vi "Single Slow IV v1.8.vi"() -> ()   [LabVIEW 2023]
uses:
  <vilib>/Utility/file.llb/Write Delimited Spreadsheet (DBL).vi
panel:
  out "Current variable":dbl=-0.010000000000000009
  in  "stop":bool
  in  "Tab Control 2":T1(tab)
  out "cRIO data plot":cluster{"Y":dbl[], "Y":dbl[]}[](graph)
  out "cRIO Plot 0":string="DC Voltage V"
  out "cRIO Plot 1":string="DC current uA"
  out "cRIO Plot 2":string="dV V"
  out "cRIO Plot 3":string="dI uA"
  out "Lockin X":cluster{"Y":dbl[], "Y":dbl[]}[](graph)
  out "Lockin Y":cluster{"Y":dbl[], "Y":dbl[]}[](graph)
  in  "Tab Control":T2(tab)
  out "Unit":string="uA"
  in  "Tab for variable":enum32{"Current", "Magnetic field"}(tab)
  in  "Delay Time s":dbl=0.1 caption="Delay Time (s)"
  in  "AO Channel":string(combo)="AO0"
  in  "current output Scale factor":dbl=1.0
  in  "Fixed current uA":dbl=2.1
  in  "Scale factor":dbl=1.0
  in  "Field Rate mT per sec":dbl=0.1 format="%#_13g"
  in  "Magnet Device Select":string(combo)="NI DAQ Controlled V to I source"
  in  "Start":dbl
  in  "Range":dbl=1.0
  in  "Step":dbl=0.01
  in  "Ramp type":string(combo)="Around origin"
  in  "Ramp up first T":bool=TRUE
  in  "cRIO Chan 0":bool=TRUE
  in  "cRIO IP":string="//172.22.11.2"
  in  "Reading Average times":i32=100
  in  "read cRIO":bool=TRUE
  in  "Scale factor3":dbl=1.0
  in  "Channel name 3":string(combo)="dI uA"
  in  "cRIO Chan 3":bool
  in  "Scale factor2":dbl=1.0
  in  "Channel name 2":string(combo)="dV V"
  in  "cRIO Chan 2":bool
  in  "Scale factor1":dbl=1.0
  in  "Channel name 1":string(combo)="DC current uA"
  in  "cRIO Chan 1":bool=TRUE
  in  "Scale factor0":dbl=0.0001
  in  "Channel name 0":string(combo)="DC Voltage V"
  in  "Lockin address 4":string
  in  "Lockin address 3":string
  in  "Lockin address 2":string="GPIB0::9::INSTR"
  in  "Lockin address 1":string="GPIB0::8::INSTR"
  in  "Lockin 4":bool
  in  "Lockin 3":bool
  in  "Lockin 2":bool
  in  "Lockin 1":bool
  in  "Use Lockin":bool
  in  "Lockin Chan name 4":string(combo)="None"
  in  "Lockin Chan name 3":string(combo)="None"
  in  "Lockin Chan name 2":string(combo)="Current mV"
  in  "Lockin Chan name 1":string(combo)="Voltage mV"
  out "DAQ_CMD_Writer endpoint":refnum<k21>="DAQ_CMD_Writer"
  out "DAQ_AI_Reader endpoint":refnum<k21>="DAQ_AI_Reader"
  in  "Lockin and field and temperature status":string="Data File time stamp 20230818-143806\nTemperature Chan1 1.218210, Chan2 0.069148\nmagnetic field InfmT\nLockin status\n"
  in  "Temp Device":string(combo)="Elsa"
  in  "Temp Chan1":string="T5"
  in  "Temp Chan2":string="T8"
  in  "Magnetic field read device":string(combo)="None"
  in  "Record Field":bool
  out "error out":errorcluster
  in  "Contour plot folder":path=path "C:/Users/gyue/Desktop/20230814 Soorya devices"
  # "NOTE:  Tab pressed below change output signal"
  # "Voltage x factor=uA"
  # "Voltage x factor=uA"
  # "Voltage x factor=actual"
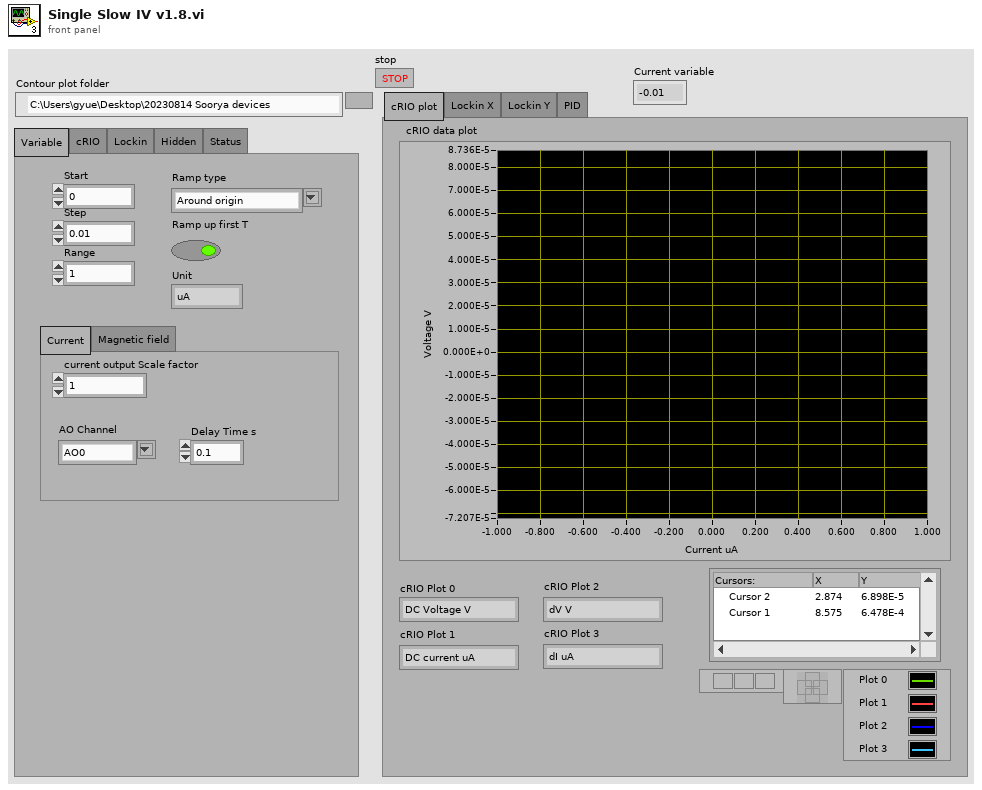
[diagram p1: front panel]
types:
  T1 = enum32{"cRIO plot", "Lockin X", "Lockin Y", "PID"}
  T2 = enum32{"Variable", "cRIO", "Lockin", "Hidden", "Status"}
  T3 = cluster{"AI0":dbl, "AI1":dbl, "AI2":dbl, "AI3":dbl}
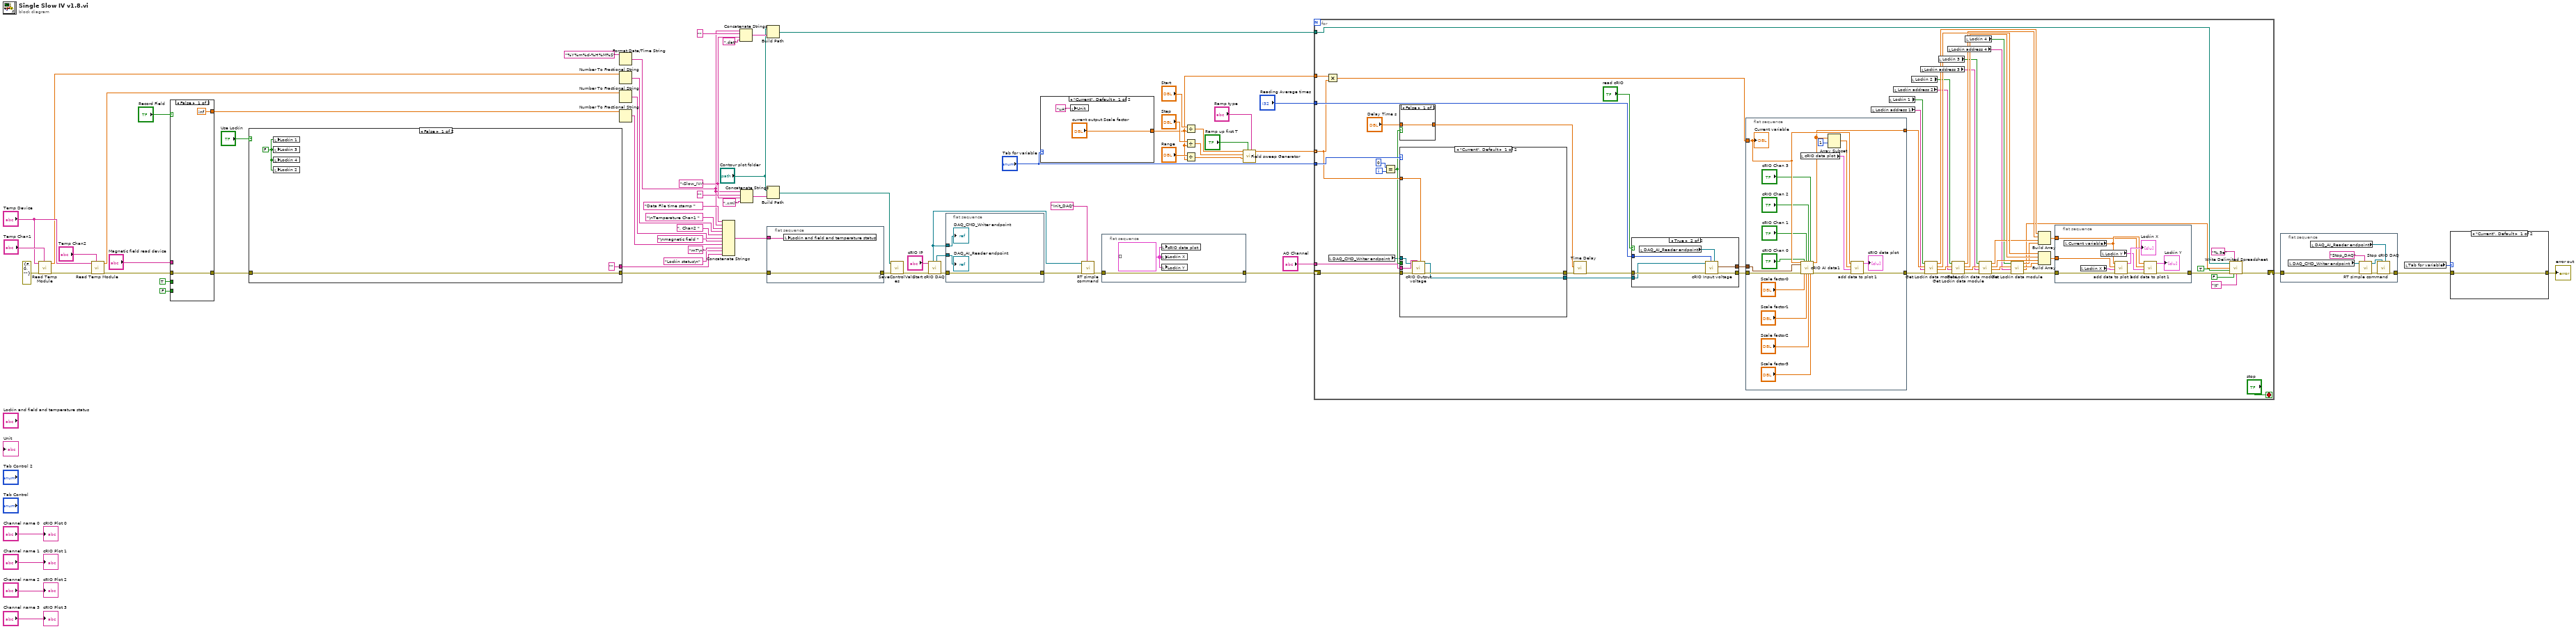
[diagram p0: block diagram]
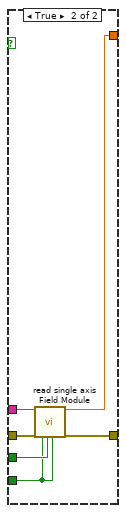
[diagram p2: hidden frame]
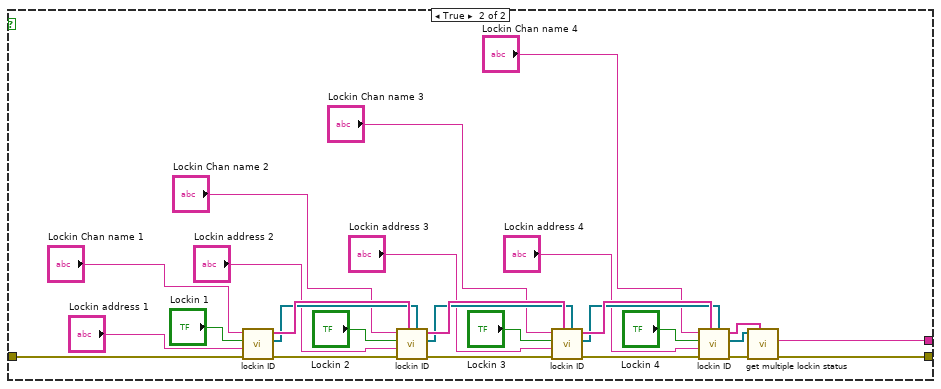
[diagram p3: hidden frame]
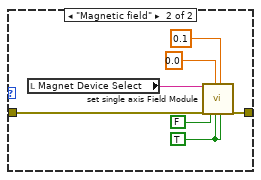
[diagram p4: hidden frame]
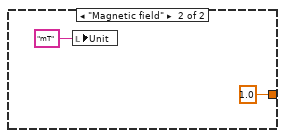
[diagram p5: hidden frame]
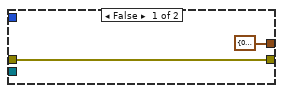
[diagram p6: hidden frame]
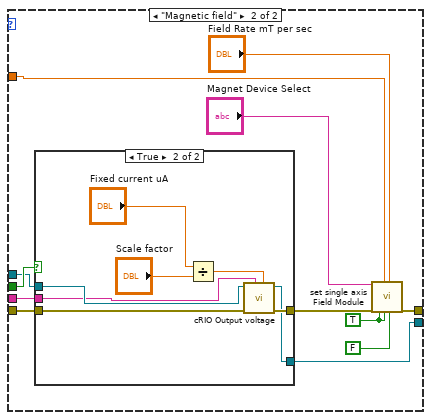
[diagram p7: hidden frame]
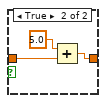
[diagram p9: hidden frame]
diagram:
  w64 = "-Slow_IV-"
  n1 = call "Read Temp Module.vi"("Temp Chan"="Temp Chan1", "error in (no error)"=errorcluster {"status"=FALSE, "code"=0, "source"=""} ("error in"), "Device"="Temp Device") -> ("error out"=w36:errorcluster, "Temperature K"=w31:dbl)  [unwired: 7 in]
  n2 = call "Read Temp Module.vi"("Temp Chan"="Temp Chan2", "error in (no error)"=w36, "Device"="Temp Device") -> ("error out"=w29:errorcluster, "Temperature K"=w30:dbl)  [unwired: 7 in]
  n3 = case shown="False" "Record Field" {
    tunnel: w29 -> [w72 w78]
    tunnel: "Magnetic field read device" -> [_ w77]
    tunnel: [inf w76] -> w27
    tunnel: TRUE ("Exec") -> [_ w75]
    tunnel: FALSE ("Init") -> [_ w74]
    tunnel: [w72 w73] -> w12
    frame False {
    }
    frame True {
      n4 = call "read single axis Field Module.vi"("Magnet Device Select"=w77, "error in (no error)"=w78, "Init"=w74, "Exec"=w75, "final"=w74) -> ("FIeld mT"=w76:dbl, "error out"=w73:errorcluster)  [unwired: 13 in]
    }
  }
  n5 = case shown="False" "Use Lockin" {
    tunnel: ["" ("Status output") w108] -> w13
    tunnel: [w81 w107] -> w11
    tunnel: w12 -> [w81 w105]
    frame False {
      w79 = FALSE ("Lockin 1")
      n6 = local write "Lockin 1"(w79) -> ()
      n7 = local write "Lockin 3"(w79) -> ()
      n8 = local write "Lockin 4"(w79) -> ()
      n9 = local write "Lockin 2"(w79) -> ()
    }
    frame True {
      n10 = call "lockin ID.vi"("error in (no error)"=w105, "Lockin address"="Lockin address 1", "Lockin on"="Lockin 1", "Lockin Chan name"="Lockin Chan name 1") -> ("error out"=w98:errorcluster, "Addresses out"=w101:refnum<visa-resource-name>[], "names out"=w102:string[])  [unwired: 5 in]
      n11 = call "lockin ID.vi"("Addresses IN"=w101, "names in"=w102, "error in (no error)"=w98, "Lockin address"="Lockin address 2", "Lockin on"="Lockin 2", "Lockin Chan name"="Lockin Chan name 2") -> ("error out"=w94:errorcluster, "Addresses out"=w95:refnum<visa-resource-name>[], "names out"=w96:string[])  [unwired: 3 in]
      n12 = call "lockin ID.vi"("Addresses IN"=w95, "names in"=w96, "error in (no error)"=w94, "Lockin address"="Lockin address 3", "Lockin on"="Lockin 3", "Lockin Chan name"="Lockin Chan name 3") -> ("error out"=w90:errorcluster, "Addresses out"=w88:refnum<visa-resource-name>[], "names out"=w89:string[])  [unwired: 3 in]
      n13 = call "lockin ID.vi"("Addresses IN"=w88, "names in"=w89, "error in (no error)"=w90, "Lockin address"="Lockin address 4", "Lockin on"="Lockin 4", "Lockin Chan name"="Lockin Chan name 4") -> ("error out"=w82:errorcluster, "Addresses out"=w83:refnum<visa-resource-name>[], "names out"=w84:string[])  [unwired: 3 in]
      n14 = call "get multiple lockin status.vi"("Device channel names"=w84, "error in (no error)"=w82, "SRS830 addresses"=w83) -> ("error out"=w107:errorcluster, "Status output"=w108:string)  [unwired: 6 in, 1 out]
    }
  }
  n15 = Format Date/Time String(time format string (%c)="%Y%m%d-%H%M%S") -> (date/time string=w23:string)  [unwired: 2 in]
  n16 = Number To Fractional String(number=w31) -> (F-format string=w20:string)  [unwired: 3 in]
  n17 = Number To Fractional String(number=w30) -> (F-format string=w19:string)  [unwired: 3 in]
  n18 = Number To Fractional String(number=w27) -> (F-format string=w17:string)  [unwired: 3 in]
  n19 = Concatenate Strings("Data File time stamp " ("string"), w23, "\nTemperature Chan1 " ("string"), w20, ", Chan2 " ("string"), w19, "\nmagnetic field " ("string"), w17, "mT\n" ("string"), "Lockin status\n" ("string"), w13) -> (w9:string)
  n20 = Concatenate Strings(w23, "" ("string"), w64, ".dat" ("string")) -> (w66:string)
  n21 = Concatenate Strings(w23, "" ("string"), w64, ".xml" ("string")) -> (w69:string)
  n22 = Build Path(base path="Contour plot folder", name or relative path=w66) -> (appended path=w51:path)
  n23 = Build Path(base path="Contour plot folder", name or relative path=w69) -> (appended path=w67:path)
  n24 = flat-sequence {
    tunnel: w11 -> [w110]
    tunnel: [w110] -> w10
    tunnel: w9 -> [w109]
    frame #0 {
      n25 = local write "Lockin and field and temperature status"(w109) -> ()
    }
  }
  n26 = call "SaveControlValues.vi"("XML File Path"=w67, "error in (no error)"=w10) -> ("error out"=w62:errorcluster)  [unwired: 8 in]
  n27 = call "Start cRIO DAQ.vi"("error in (no error)"=w62, "cRIO IP"="cRIO IP") -> ("error out"=w6:errorcluster, "DAQ_AI_Reader endpoint"=w50:refnum<k21>, "DAQ_CMD_Writer endpoint"=w3:refnum<k21>)  [unwired: 7 in]
  n28 = flat-sequence {
    tunnel: w3 -> [w113]
    tunnel: w50 -> [w112]
    tunnel: w6 -> [w111]
    tunnel: [w111] -> w5
    frame #0 {
      "DAQ_CMD_Writer endpoint" <- w113
      "DAQ_AI_Reader endpoint" <- w112
    }
  }
  n29 = case shown="\"Current\", Default" "Tab for variable" {
    tunnel: ["current output Scale factor" 1.0 ("current output Scale factor")] -> w40
    frame "Current", Default {
      n30 = local write "Unit"("uA" ("Unit")) -> ()
    }
    frame "Magnetic field" {
      n31 = local write "Unit"("mT" ("Unit")) -> ()
    }
  }
  n32 = call "RT simple command.vi"("Command"="Init_DAQ", "error in (no error)"=w5, "DAQ_CMD_Writer endpoint"=w3) -> ("error out"=w4:errorcluster)  [unwired: 7 in, 1 out]
  n33 = flat-sequence {
    tunnel: w4 -> [w119]
    tunnel: [w119] -> w7
    frame #0 {
      w118 = cluster{dbl[], dbl[]}[] [] ("appended array")
      n34 = local write "cRIO data plot"(w118) -> ()
      n35 = local write "Lockin X"(w118) -> ()
      n36 = local write "Lockin Y"(w118) -> ()
    }
  }
  n37 = Divide(x="Start", y=w40) -> (x/y=w42:dbl)
  n38 = Divide(x="Step", y=w40) -> (x/y=w55:dbl)
  n39 = Divide(x="Range", y=w40) -> (x/y=w54:dbl)
  n40 = call "Field sweep Generator.vi"("Ramp type"="Ramp type", "Ramp up first T"="Ramp up first T", "Field Radius"=w54, "Field step"=w55, "Field Origin"=w42) -> ("output array"=w52:dbl[])  [unwired: 6 in]
  n41 = for {
    tunnel: "AO Channel" -> [w159]
    tunnel: w52 -> [w160] mode=indexing
    tunnel: w51 -> [w174]
    tunnel: "Reading Average times" -> [w167]
    tunnel: "Tab for variable" -> [w161]
    tunnel: w40 -> [w155]
    shift-right: [w168] -> w1
    shift-left: w7 -> [w153]
    i -> [w165]
    stop <- "stop" stop-if-true
    n42 = Multiply(x=w155, y=w160) -> (x*y=w151:dbl)
    n43 = local read "DAQ_CMD_Writer endpoint"() -> (w120:refnum<k21>)
    n44 = Equal?(x=0, y=w165) -> (x = y?=w156:bool)
    n45 = case shown="False" w156 {
      tunnel: "Delay Time s" -> [w239 w240]
      tunnel: [w239 w242] -> w162
      frame False {
      }
      frame True {
        n46 = Add(x=5.0 ("Delay Time s"), y=w240) -> (x+y=w242:dbl)
      }
    }
    n47 = case shown="\"Current\", Default" w161 {
      tunnel: w160 -> [w216 w220]
      tunnel: w159 -> [w215 w224]
      tunnel: w153 -> [w214 w227]
      tunnel: w120 -> [w213 w226]
      tunnel: [w212 w222] -> w158
      tunnel: [w211 w225] -> w157
      tunnel: w156 -> [_ w228]
      frame "Current", Default {
        n48 = call "cRIO Output voltage.vi"("Voltage"=w216, "AO Channel"=w215, "error in (no error)"=w214, "DAQ_CMD_Writer endpoint"=w213) -> ("error out"=w212:errorcluster, "DAQ_CMD_Writer endpoint out"=w211:refnum<k21>)  [unwired: 6 in]
      }
      frame "Magnetic field" {
        w218 = TRUE ("Init")
        n49 = case shown="True" w228 {
          tunnel: w227 -> [w229 w238]
          tunnel: [w229 w237] -> w223
          tunnel: w226 -> [w230 w236]
          tunnel: [w230 w235] -> w225
          tunnel: w224 -> [_ w234]
          frame False {
          }
          frame True {
            n50 = Divide(x="Fixed current uA", y="Scale factor") -> (x/y=w232:dbl)
            n51 = call "cRIO Output voltage.vi"("Voltage"=w232, "AO Channel"=w234, "error in (no error)"=w238, "DAQ_CMD_Writer endpoint"=w236) -> ("error out"=w237:errorcluster, "DAQ_CMD_Writer endpoint out"=w235:refnum<k21>)  [unwired: 6 in]
          }
        }
        n52 = call "set single axis Field Module.vi"("Field Device Select"="Magnet Device Select", "error in (no error)"=w223, "Init"=w218, "Field Target mT or dBm"=w220, "Exec"=w218, "Field Rate mT per sec"="Field Rate mT per sec", "final"=FALSE ("Exec")) -> ("error out"=w222:errorcluster)  [unwired: 12 in]
      }
    }
    n53 = call "Time Delay"("error in (no error)"=w158, "Delay Time (s)"=w162) -> ("error out"=w170:errorcluster)  [unwired: 9 in]
    n54 = case shown="True" "read cRIO" {
      tunnel: w170 -> [w204 w210]
      tunnel: [w204 w209] -> w149
      tunnel: w167 -> [_ w208]
      tunnel: w157 -> [_ w207]
      tunnel: [T3 {"AI0"=0.0, "AI1"=0.0, "AI2"=0.0, "AI3"=0.0} ("output cluster") w206] -> w150
      frame False {
      }
      frame True {
        n55 = local read "DAQ_AI_Reader endpoint"() -> (w205:refnum<k21>)
        n56 = call "cRIO Input voltage.vi"("DAQ_AI_Reader endpoint"=w205, "Average"=w208, "error in (no error)"=w210, "DAQ_CMD_Writer endpoint"=w207) -> ("error out"=w209:errorcluster, "output cluster"=w206:T3)  [unwired: 5 in, 1 out]
      }
    }
    n57 = flat-sequence {
      tunnel: w151 -> [w201]
      tunnel: w150 -> [w200]
      tunnel: w149 -> [w199]
      tunnel: [w192] -> w148
      tunnel: [w187] -> w147
      frame #0 {
        n58 = local read "cRIO data plot"() -> (w202:cluster{"Y":dbl[], "Y":dbl[]}[])
        n59 = call "cRIO AI data1.vi"("I"=w201, "Input cluster"=w200, "error in (no error)"=w199, "Chan 0"="cRIO Chan 0", "Scale factor0"="Scale factor0", "Chan 1"="cRIO Chan 1", "Scale factor1"="Scale factor1", "Chan 2"="cRIO Chan 2", "Scale factor2"="Scale factor2", "Chan 3"="cRIO Chan 3", "Scale factor3"="Scale factor3") -> ("Output data"=w187:dbl[], "error out"=w193:errorcluster)  [unwired: 7 in]
        n60 = Array Subset(array=w187, index=1) -> (w185:dbl[])  [unwired: 1 in]
        n61 = call "add data to plot 1.vi"("error in (no error)"=w193, "Input graph"=w202, "Input Y array"=w185, "x"=w201) -> ("error in (no error) 2"=w192:errorcluster, "Output graph"=→"cRIO data plot":cluster{dbl[], dbl[]}[])  [unwired: 6 in]
        "Current variable" <- w201
      }
    }
    n62 = local read "Lockin address 1"() -> (w141:string)
    n63 = local read "Lockin 1"() -> (w152:bool)
    n64 = local read "Lockin address 2"() -> (w138:string)
    n65 = local read "Lockin 2"() -> (w140:bool)
    n66 = local read "Lockin address 3"() -> (w131:string)
    n67 = call "Get Lockin data module.vi"("error in (no error)"=w148, "Lockin address 1"=w141, "Output data in"=w147, "Lockin 1"=w152) -> ("error out"=w137:errorcluster, "Output data out"=w139:dbl[], "X mV"=w145:dbl, "Y mV"=w143:dbl)  [unwired: 4 in]
    n68 = local read "Lockin 3"() -> (w134:bool)
    n69 = local read "Lockin address 4"() -> (w125:string)
    n70 = call "Get Lockin data module.vi"("error in (no error)"=w137, "Lockin address 1"=w138, "Output data in"=w139, "Lockin 1"=w140) -> ("error out"=w132:errorcluster, "Output data out"=w133:dbl[], "X mV"=w135:dbl, "Y mV"=w136:dbl)  [unwired: 4 in]
    n71 = local read "Lockin 4"() -> (w128:bool)
    n72 = call "Get Lockin data module.vi"("error in (no error)"=w132, "Lockin address 1"=w131, "Output data in"=w133, "Lockin 1"=w134) -> ("error out"=w126:errorcluster, "Output data out"=w127:dbl[], "X mV"=w129:dbl, "Y mV"=w130:dbl)  [unwired: 4 in]
    n73 = call "Get Lockin data module.vi"("error in (no error)"=w126, "Lockin address 1"=w125, "Output data in"=w127, "Lockin 1"=w128) -> ("error out"=w122:errorcluster, "Output data out"=w121:dbl[], "X mV"=w123:dbl, "Y mV"=w124:dbl)  [unwired: 4 in]
    n74 = Build Array(w143, w136, w130, w124) -> (w142:dbl[])
    n75 = Build Array(w145, w135, w129, w123) -> (w144:dbl[])
    n76 = flat-sequence {
      tunnel: w122 -> [w181]
      tunnel: [w179] -> w146
      tunnel: w144 -> [w182]
      tunnel: w142 -> [w175]
      frame #0 {
        n77 = local read "Current variable"() -> (w178:dbl)
        n78 = local read "Lockin X"() -> (w184:cluster{"Y":dbl[], "Y":dbl[]}[])
        n79 = local read "Lockin Y"() -> (w177:cluster{"Y":dbl[], "Y":dbl[]}[])
        n80 = call "add data to plot 1.vi"("error in (no error)"=w181, "Input graph"=w184, "Input Y array"=w182, "x"=w178) -> ("error in (no error) 2"=w180:errorcluster, "Output graph"=→"Lockin X":cluster{dbl[], dbl[]}[])  [unwired: 6 in]
        n81 = call "add data to plot 1.vi"("error in (no error)"=w180, "Input graph"=w177, "Input Y array"=w175, "x"=w178) -> ("error in (no error) 2"=w179:errorcluster, "Output graph"=→"Lockin Y":cluster{dbl[], dbl[]}[])  [unwired: 6 in]
      }
    }
    n82 = call-poly <vilib>:"Write Delimited Spreadsheet.vi"("file path (dialog if empty)"=w174, "format (%.3f)"="%.9e", "1D data"=w121, "append to file? (new file:F)"=TRUE, "error in (no error)"=w146, "transpose? (no:F)"=FALSE, "delimiter (\\t)"="\t" ("delimiter (\\t)")) -> ("error out"=w168:errorcluster)  [unwired: 7 in, 1 out]
  }
  n83 = flat-sequence {
    tunnel: [w249] -> w38
    tunnel: w1 -> [w244]
    frame #0 {
      n84 = local read "DAQ_CMD_Writer endpoint"() -> (w245:refnum<k21>)
      n85 = local read "DAQ_AI_Reader endpoint"() -> (w248:refnum<k21>)
      n86 = call "RT simple command.vi"("Command"="Stop_DAQ", "error in (no error)"=w244, "DAQ_CMD_Writer endpoint"=w245) -> ("error out"=w243:errorcluster, "DAQ_CMD_Writer endpoint out"=w246:refnum<k21>)  [unwired: 7 in]
      n87 = call "Stop cRIO DAQ.vi"("DAQ_AI_Reader endpoint"=w248, "DAQ_CMD_Writer endpoint"=w246, "error in (no error)"=w243) -> ("error out"=w249:errorcluster)  [unwired: 8 in]
    }
  }
  n88 = local read "Tab for variable"() -> (w39:enum32{"Current", "Magnetic field"})
  n89 = case shown="\"Current\", Default" w39 {
    tunnel: w38 -> [w250 w254]
    tunnel: [w250 w253] -> w37
    frame "Current", Default {
    }
    frame "Magnetic field" {
      w251 = TRUE ("Exec")
      n90 = local read "Magnet Device Select"() -> (w257:string)
      n91 = call "set single axis Field Module.vi"("Field Device Select"=w257, "error in (no error)"=w254, "Init"=FALSE, "Field Target mT or dBm"=0.0 ("Field Target mT"), "Exec"=w251, "Field Rate mT per sec"=0.1, "final"=w251) -> ("error out"=w253:errorcluster)  [unwired: 12 in]
    }
  }
  "error out" <- w37
  "cRIO Plot 0" <- "Channel name 0"
  "cRIO Plot 1" <- "Channel name 1"
  "cRIO Plot 2" <- "Channel name 2"
  "cRIO Plot 3" <- "Channel name 3"
